vi "TranslateRequestTopic.vi"(2 "String w/o Tag":string, 3 "Registered":T2[](array[typedef])) -> (0 "XML":string, 1 "New Sub":T1)   [LabVIEW 2012]
doc: "Returns the port or if the port already exists, make up a new one and then add that to the publisher queue"
uses:
  <userlib>/ROS for LabVIEW Software/ROS/Code/SubVIs/_ROSControl.ctl
  <userlib>/ROS for LabVIEW Software/ROS/Code/SubVIs/_ROSDirection.ctl
panel:
  out "topic port":u16
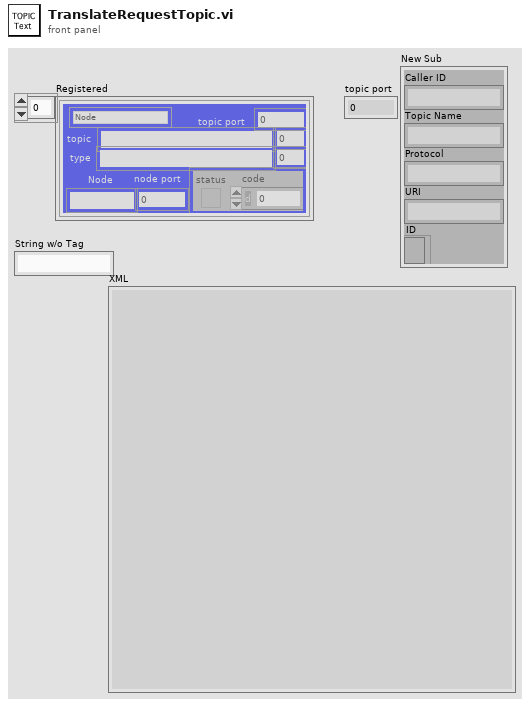
[diagram p1: front panel]
types:
  T1 = cluster{"Caller ID":string, "Topic Name":string, "Protocol":string, "URI":string, "ID":refnum<k5>}
  T2 = typedef "_ROSControl.ctl" = cluster{"topic port":u16, "Node":string, "topic":string, "type":string, "node port":u16, "error ":errorcluster, "Direction":T3, "Update (ms)":u16, "FIFO size":u16}
  T3 = typedef "_ROSDirection.ctl" = enum16{"Node", "Publisher", "Subscriber", "ServiceClient", "ServiceProvider"}
  T4 = enum16{"http://IP:port", "http://IP", "IP:port", "IP only"}
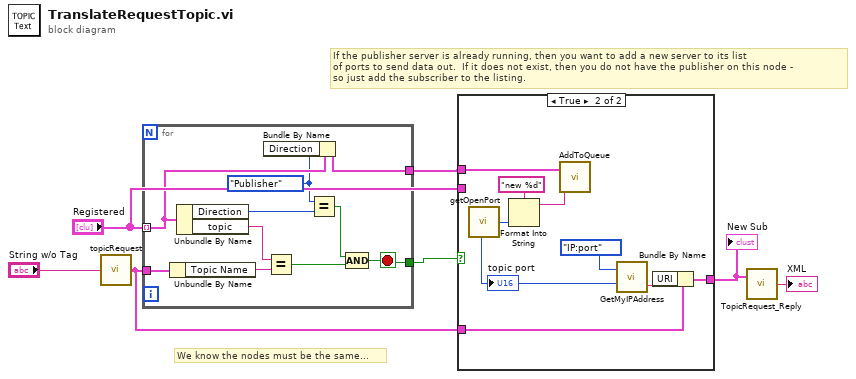
[diagram p0: block diagram]
diagram:
  # "If the publisher server is already running, then you want to add a new server to its list\nof ports to send data out.  If it does not exist, then you do not have the publisher on this node - \nso just add the subscriber to the listing."
  # "We know the nodes must be the same..."
  n1 = call <userlib>:"topicRequest.vi"("XML"="String w/o Tag") -> ("Subscriber"=w6:T1)
  n2 = for {
    tunnel: "Registered" -> [w10] mode=indexing
    tunnel: w6 -> [w17]
    tunnel: [w11] -> w3
    tunnel: [w8] -> w1
    stop <- w11 stop-if-true
    w9 = _ROSDirection."Publisher" ("x")
    n3 = Unbundle By Name(w17) -> ("Topic Name"=w16:string)
    n4 = Unbundle By Name(w10) -> ("Direction"=w14:T3, "topic"=w15:string)
    n5 = Bundle By Name(cluster=w10, "Direction"=w9) -> (w8:T2)
    n6 = Equal?(x=w15, y=w16) -> (x = y?=w12:bool)
    n7 = Equal?(x=w9, y=w14) -> (x = y?=w13:bool)
    n8 = Compound Arithmetic op=AND(w13, w12) -> (w11:bool)
  }
  n9 = case shown="True" w3 {
    tunnel: w6 -> [w18 w20]
    tunnel: [w18 w19] -> w5
    tunnel: "Registered" -> [_ _]
    tunnel: w1 -> [_ w22]
    frame False {
    }
    frame True {
      n10 = call <userlib>:"getOpenPort.vi"() -> ("port"=w23:u16)
      "topic port" <- w23
      n11 = Format Into String(format string="new %d", w23) -> (resulting string=w21:string)  [unwired: 2 in, 1 out]
      n12 = call <userlib>:"AddToQueue.vi"("Cmd"=w21, "ROS"=w22) -> ()  [unwired: 3 in, 1 out]
      n13 = call <userlib>:"GetMyIPAddress.vi"("Port"=w23, "Format"=T4."IP:port") -> ("URI"=w25:string)  [unwired: 1 out]
      n14 = Bundle By Name(cluster=w20, "URI"=w25) -> (w19:T1)
    }
  }
  "New Sub" <- w5
  n15 = call <userlib>:"TopicRequest_Reply.vi"("Subscriber"=w5) -> ("XML"=→"XML":string)  [unwired: 1 in]
